vi "KundtsTube.vi"() -> ()   [LabVIEW 2014]
panel:
  out "Gain out":dbl[](array[numeric])
  in  "Parameters":T1={"Sampling Rate (Hz)"=100000.0, "# of Samples"=1000.0}
  out "RMS":dbl
  out "Waveform Graph":dynamicdata(graph)
  in  "stop":bool
  in  "Amplitude (V)":dbl
  out "XY Graph":cluster{dbl[], dbl[]}(graph)
  in  "Tab Control":enum32{"Sweep", "Single"}(tab)
  in  "Dwell Time, sec":dbl
  in  "Frequency (Hz)":dbl
  in  "Input Values":T2
  # "A single frequency is played"
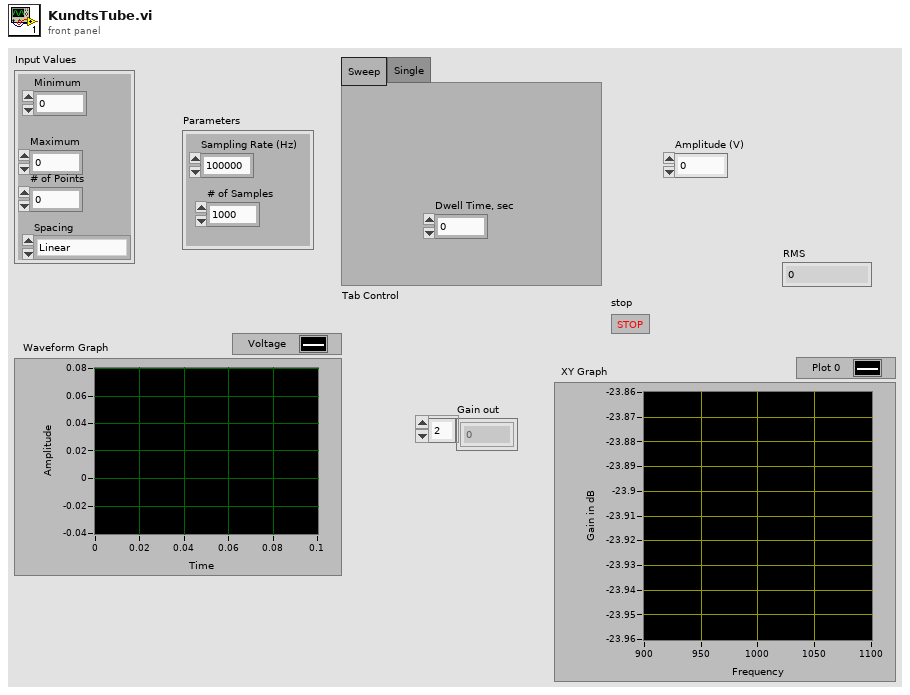
[diagram p1: front panel]
types:
  T1 = cluster{"Sampling Rate (Hz)":dbl, "# of Samples":dbl}
  T2 = cluster{"Minimum":i32, "Maximum":i32, "# of Points":i32, "Spacing":enum16{"Linear", "Logarithmic"}}
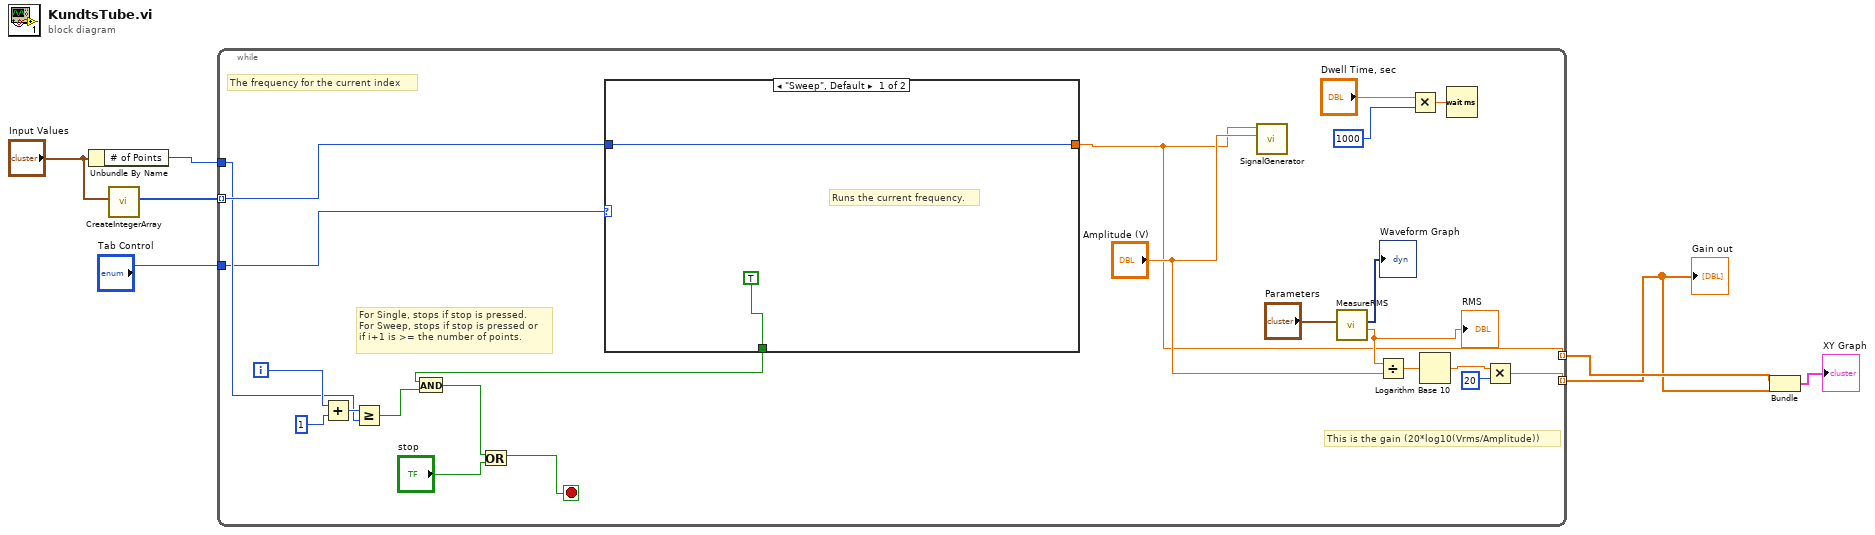
[diagram p0: block diagram]
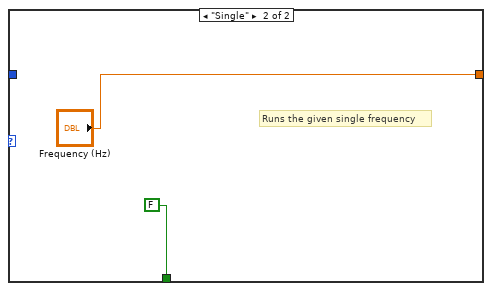
[diagram p2: hidden frame]
diagram:
  n1 = Unbundle By Name("Input Values") -> ("# of Points"=w4:i32)
  n2 = call "CreateIntegerArray.vi"("Input Values"="Input Values") -> ("Output Array"=w5:i32[])  [unwired: 10 in]
  n3 = while {
    tunnel: "Tab Control" -> [w11]
    tunnel: w5 -> [w30] mode=indexing
    tunnel: w4 -> [w24]
    tunnel: [w13] -> w2 mode=indexing
    tunnel: [w12] -> w3 mode=indexing
    i -> [w25]
    stop <- w28 stop-if-true
    # "For Single, stops if stop is pressed.\nFor Sweep, stops if stop is pressed or\nif i+1 is >= the number of points."
    # "The frequency for the current index"
    # "This is the gain (20*log10(Vrms/Amplitude))"
    n4 = Add(x=w25, y=1) -> (x+y=w27:i32)
    n5 = Greater Or Equal?(x=w27, y=w24) -> (x >= y?=w9:bool)
    n6 = case shown="\"Sweep\", Default" w11 {
      tunnel: [w32 "Frequency (Hz)"] -> w12
      tunnel: w30 -> [w32 _]
      tunnel: [TRUE FALSE] -> w10
      frame "Sweep", Default {
        # "Runs the current frequency."
      }
      frame "Single" {
        # "Runs the given single frequency"
      }
    }
    n7 = And(x=w10, y=w9) -> (x .and. y?=w8:bool)
    n8 = Or(x=w8, y="stop") -> (x .or. y?=w28:bool)
    n9 = call "SignalGenerator.vi"("Amplitude (V)"="Amplitude (V)", "Frequency (Hz)"=w12) -> ()  [unwired: 10 in]
    n10 = call "MeasureRMS.vi"("Parameters"="Parameters") -> ("RMS"=w19:dbl, "Waveform Graph"=→"Waveform Graph":dynamicdata)  [unwired: 9 in]
    "RMS" <- w19
    n11 = Divide(x=w19, y="Amplitude (V)") -> (x/y=w21:dbl)
    n12 = Multiply(x="Dwell Time, sec", y=1000) -> (x*y=w22:dbl)
    n13 = Logarithm Base 10(1:w21) -> (0:w16:dbl)
    n14 = Wait (ms)(milliseconds to wait=w22) -> ()  [unwired: 1 out]
    n15 = Multiply(x=w16, y=20) -> (x*y=w13:dbl)
  }
  "Gain out" <- w2
  n16 = Bundle(w3, w2) -> (→"XY Graph":cluster{dbl[], dbl[]})  [unwired: 1 in]
